vi "date_filename.vi"() -> (2 "Path":path, 3 "result string":string)   [LabVIEW 2020]
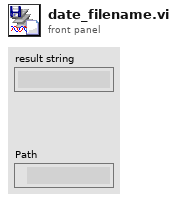
[diagram p1: front panel]
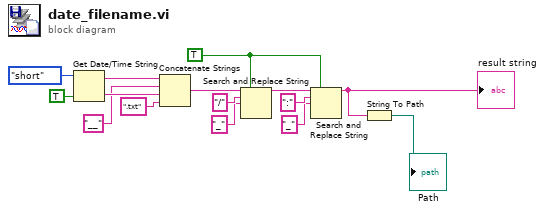
[diagram p0: block diagram]
diagram:
  w5 = TRUE ("replace all? (F)")
  n1 = Get Date/Time String(date format (0)=enum16{"short", "long", "abbreviated"}."short", want seconds? (F)=TRUE) -> (date string=w13:string, time string=w4:string)  [unwired: 1 in]
  n2 = Concatenate Strings(w13, "__" ("string"), w4, ".txt") -> (w11:string)
  n3 = Search and Replace String(replace all?=w5, input string=w11, search string="/", replace string="_" ("replace string (\"\")")) -> (result string=w8:string)  [unwired: 4 in, 3 out]
  n4 = Search and Replace String(replace all?=w5, input string=w8, search string=":", replace string="_" ("replace string (\"\")")) -> (result string=w1:string)  [unwired: 4 in, 3 out]
  "result string" <- w1
  n5 = String To Path(string=w1) -> (path=→"Path":path)
